vi "Call Stop.vi"(6 "Diagnostics Queue in":refnum<queue>, 7 "Host Resources":T10, 8 "error in (no error)":errorcluster, 11 "Hardware Configuration in":T1) -> (0 "error out":errorcluster, 3 "Hardware Configuration out":T1)   [LabVIEW 2021, in "Acquisition.lvlib"]
uses:
  Acquisition.lvlib
  support/Message Queue/Message Cluster.ctl
  Host Resources.ctl
  Host Software Package.ctl
  Host IO Resource.ctl
  Hardware Configuration.ctl
  Channel Settings.ctl
  IO Device.ctl
  Sensor Type.ctl
  Interval Timer/Repeat Interval.ctl
  Interval Timer/Interval Length.ctl
  Interval Timer/Interval Token.ctl
  IO Context.ctl
  IO API.ctl
  API Call.ctl
  support/Message Queue/Message Queue.lvlib
  Interval Timer/Interval Timer.lvlib
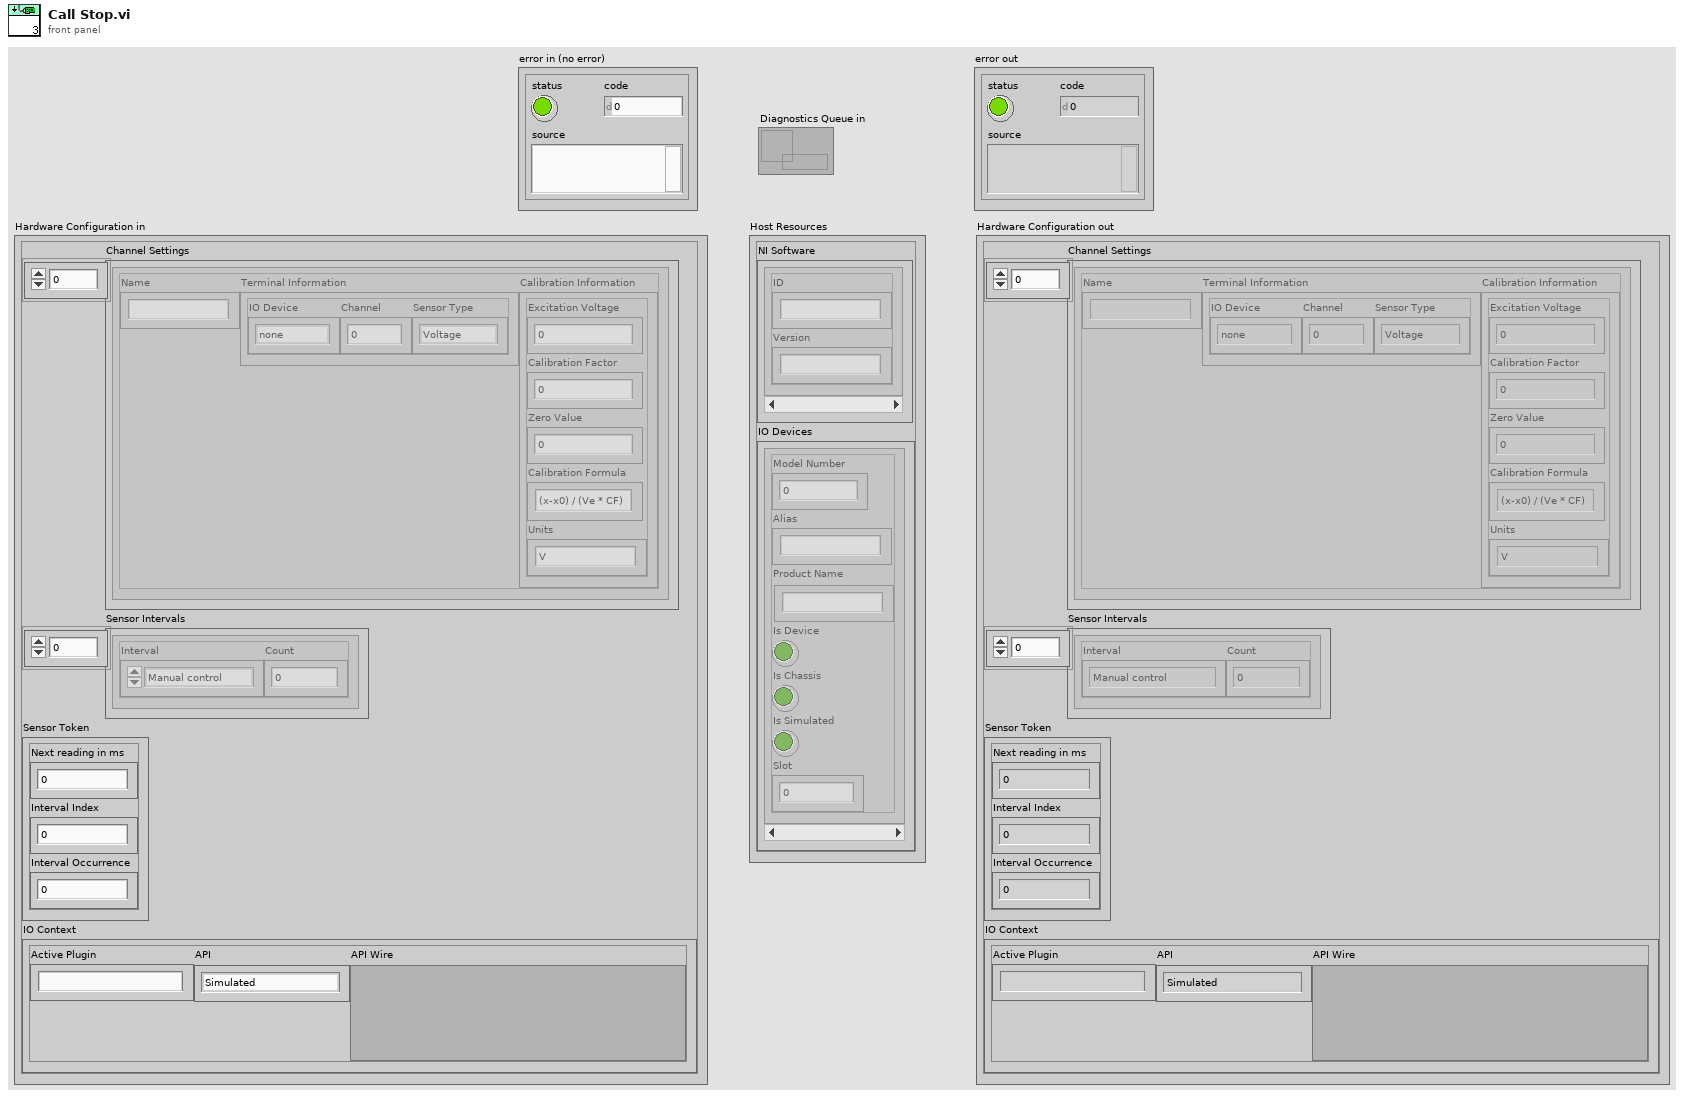
[diagram p1: front panel]
types:
  T1 = typedef "Acquisition.lvlib/Hardware Configuration.ctl" = cluster{"Channel Settings":T2[], "Sensor Intervals":T5[], "Sensor Token":T7, "IO Context":T8}
  T2 = typedef "Acquisition.lvlib/Channel Settings.ctl" = cluster{"Name":string, "Terminal Information":cluster{"IO Device":T3, "Channel":i32, "Sensor Type":T4}, "Calibration Information":cluster{"Excitation Voltage":dbl, "Calibration Factor":dbl, "Zero Value":dbl, "Calibration Formula":string, "Units":string}}
  T3 = typedef "Acquisition.lvlib/IO Device.ctl" = enum16{"none", "9219", "9401"}
  T4 = typedef "Acquisition.lvlib/Sensor Type.ctl" = enum16{"Voltage", "Load", "Pressure", "Encoder"}
  T5 = typedef "Interval Timer.lvlib/Repeat Interval.ctl" = cluster{"Interval":T6, "Count":i32}
  T6 = typedef "Interval Timer.lvlib/Interval Length.ctl" = enum16{"Manual control", "1 second", "10 seconds", "30 seconds", "60 seconds", "600 seconds", "1200 seconds", "3600 seconds"}
  T7 = typedef "Interval Timer.lvlib/Interval Token.ctl" = cluster{"Next reading in ms":u32, "Interval Index":i32, "Interval Occurrence":i32}
  T8 = typedef "Acquisition.lvlib/IO Context.ctl" = cluster{"Active Plugin":string, "API":T9, "API Wire":variant}
  T9 = typedef "Acquisition.lvlib/IO API.ctl" = enum16{"Simulated", "DAQmx"}
  T10 = typedef "Acquisition.lvlib/Host Resources.ctl" = cluster{"NI Software":T11[], "IO Devices":T12[]}
  T11 = typedef "Acquisition.lvlib/Host Software Package.ctl" = cluster{"ID":string, "Version":string}
  T12 = typedef "Acquisition.lvlib/Host IO Resource.ctl" = cluster{"Model Number":u32, "Alias":string, "Product Name":string, "Is Device":bool, "Is Chassis":bool, "Is Simulated":bool, "Slot":i32}
  T13 = typedef "Acquisition.lvlib/API Call.ctl" = enum16{"On Start", "Acquire", "On Stop", "Preview"}
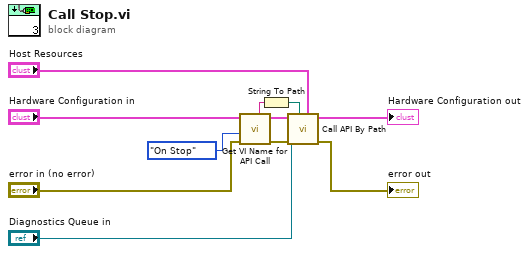
[diagram p0: block diagram]
diagram:
  n1 = call "Get VI Name for API Call.vi"("error in"="error in (no error)", "API Call"=API_Call."On Stop", "Hardware Configuration in"="Hardware Configuration in") -> ("error out"=w4:errorcluster, "Hardware Configuration out"=w1:T1, "VI Name"=w6:string)  [unwired: 6 in]
  n2 = String To Path(string=w6) -> (path=w7:path)
  n3 = call "Call API By Path.vi"("Host Resources"="Host Resources", "vi path"=w7, "error in"=w4, "Diagnostics Queue"="Diagnostics Queue in", "Hardware Configuration in"=w1) -> ("error out"=→"error out":errorcluster, "Hardware Configuration out"=→"Hardware Configuration out":T1)  [unwired: 4 in, 1 out]
